vi "WriteCmdOut.vi"(0 "Connections In":T1(array[cluster]), 2 "Log in":T2[](array[typedef]), 3 "Err in":string, 4 "data":string) -> (5 "Connections Out":T1(array[cluster]), 6 "Log out":T2[](array[typedef]), 7 "Err out":string)   [LabVIEW 2012]
uses:
  <userlib>/ROSforLV/ROS/Code/Console/Servers/ServerSubs/ROSLog.ctl
  <userlib>/ROSforLV/ROS/Code/_ROSDefinition.vi
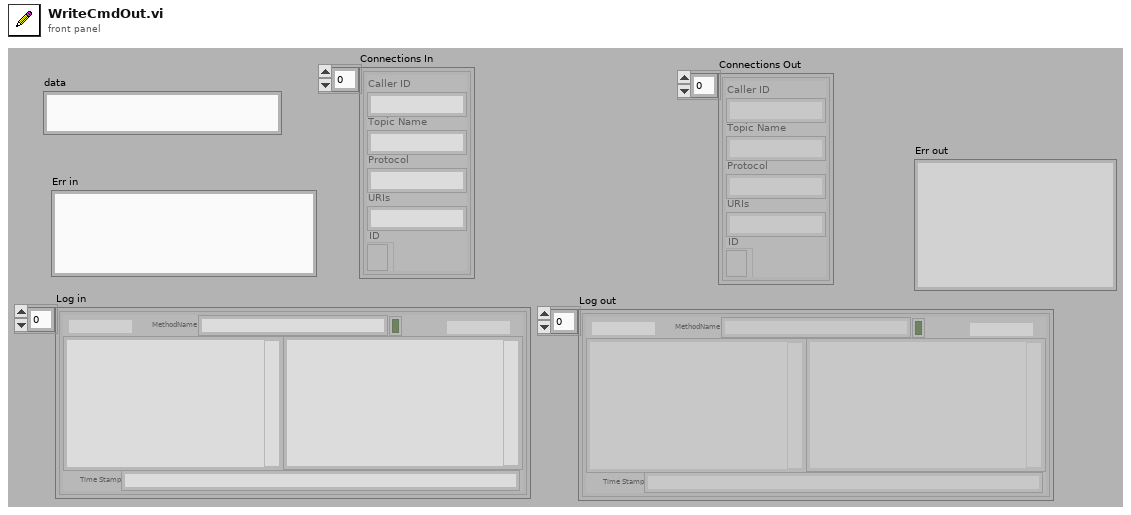
[diagram p1: front panel]
types:
  T1 = cluster{"Caller ID":string, "Topic Name":string, "Protocol":string, "URIs":string, "ID":refnum<k5>}[]
  T2 = typedef "ROSLog.ctl" = cluster{"Sent":string, "Reply":string, "MethodName":string, "success":bool, "Dir1":string, "Dir2":string, "Time Stamp":string}
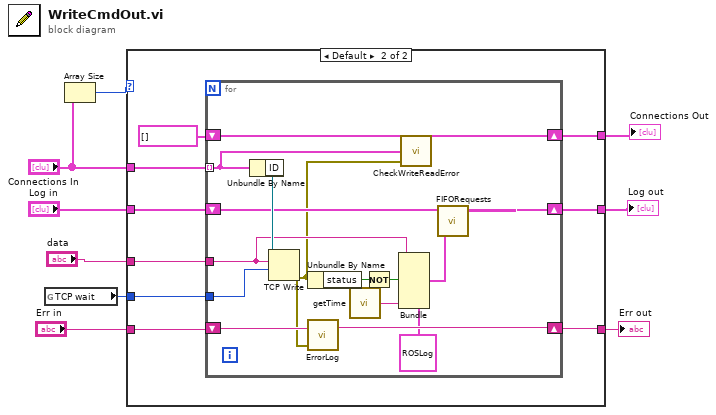
[diagram p0: block diagram]
diagram:
  n1 = global read "_ROSDefinition.vi" "TCP wait"() -> (w1:i32)
  n2 = Array Size(array="Connections In") -> (size(s)=w4:i32)
  n3 = case shown="Default" w4 {
    tunnel: [w12 w21] -> w9
    tunnel: "Log in" -> [w12 w20]
    tunnel: "Err in" -> [w11 w19]
    tunnel: [w11 w18] -> w6
    tunnel: "Connections In" -> [w10 w17]
    tunnel: "data" -> [_ w16]
    tunnel: [w10 w14] -> w2
    tunnel: w1 -> [_ w13]
    frame 0 {
    }
    frame Default {
      n4 = for {
        shift-right: [w37] -> w18
        shift-left: w19 -> [w36]
        shift-right: [w28] -> w21
        shift-left: w20 -> [w29]
        tunnel: w17 -> [w27] mode=indexing
        tunnel: w16 -> [w30]
        shift-right: [w24] -> w14
        shift-left: T1 [] -> [w23]
        tunnel: w13 -> [w22]
        n5 = Unbundle By Name(w27) -> ("ID"=w35:refnum<k5>)
        n6 = TCP Write(connection ID=w35, data in=w30, 9:w22) -> (error out=w25:errorcluster)  [unwired: 1 in, 2 out]
        n7 = Unbundle By Name(w25) -> ("status"=w32:bool)
        n8 = call <userlib>:"ErrorLog.vi"("error in"=w25, "String in"=w36) -> ("String out"=w37:string)  [unwired: 1 in, 1 out]
        n9 = call <userlib>:"getTime.vi"() -> ("Current Time"=w34:string)  [unwired: 1 in]
        n10 = Not(x=w32) -> (.not. x?=w31:bool)
        n11 = Bundle(cluster=T2 {"Sent"="", "Reply"="", "MethodName"="write", "success"=FALSE, "Dir1"="To ROS", "Dir2"="From ROS", "Time Stamp"=""} ("Log"), "Sent"=w30, "success"=w31, "Time Stamp"=w34) -> (w33:T2)  [unwired: 4 in]
        n12 = call <userlib>:"CheckWriteReadError.vi"("error"=w25, "Subscriber in"=w27, "Connections in"=w23) -> ("Connections out"=w24:T1)
        n13 = call <userlib>:"FIFORequests.vi"("Log"=w33, "Requests in"=w29) -> ("Requests out"=w28:T2[])  [unwired: 1 in]
      }
    }
  }
  "Log out" <- w9
  "Err out" <- w6
  "Connections Out" <- w2
